vi "Release Mapped Memory Access.vi"   [LabVIEW 2020, in "image.lvlib"]
doc: "Release the Mapped Memory Access. This will invalidate the guarantee that the image's underlying memory is locked and its layout is fixed."
uses:
  image.lvlib
  Mapped Memory Access Image Greyscale/Mapped Memory Access Image Greyscale.lvclass
  Mapped Memory Access Image ARGB/Mapped Memory Access Image ARGB.lvclass
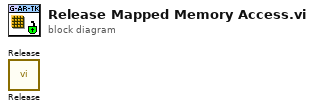
[diagram p0: block diagram]
diagram:
  n1 = call "Release.vi"() -> ()  [unwired: 10 in, 2 out]
  n2 = call "Release.vi"() -> ()  [unwired: 10 in, 2 out]
